vi "RGB Brightness.vi"(9 "Red":u8, 10 "Green":u8, 11 "Blue":u8) -> (3 "Brightness":u8)   [LabVIEW 2013]
panel:
  in  "Weights":cluster{"Green":u32, "Blue":u32, "Red":u32}={"Green"=587, "Blue"=114, "Red"=299}
  # "Weight Constants are from\nhttp://www.had2know.com/technology/color-contrast-calculator-web-design.html"
  # "Red: 299"
  # "Green: 587"
  # "Blue: 114"
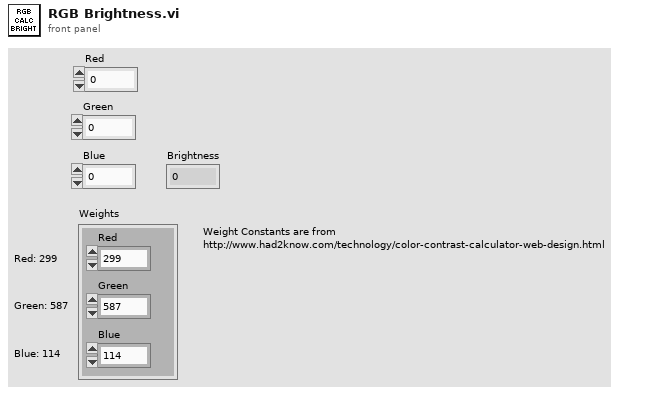
[diagram p1: front panel]
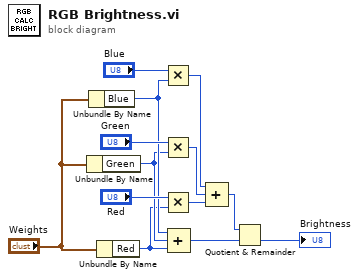
[diagram p0: block diagram]
diagram:
  n1 = Unbundle By Name("Weights") -> ("Green"=w2:u32)
  n2 = Unbundle By Name("Weights") -> ("Blue"=w3:u32)
  n3 = Unbundle By Name("Weights") -> ("Red"=w1:u32)
  n4 = Multiply(x="Blue", y=w3) -> (x*y=w9:u32)
  n5 = Multiply(x="Green", y=w2) -> (x*y=w8:u32)
  n6 = Multiply(x="Red", y=w1) -> (x*y=w7:u32)
  n7 = Compound Arithmetic op=ADD(w3, w2, w1) -> (w5:u32)
  n8 = Compound Arithmetic op=ADD(w9, w8, w7) -> (w6:u32)
  n9 = Quotient & Remainder(x=w6, y=w5) -> (floor(x/y)=→"Brightness":u32)  [unwired: 1 out]
